vi "Sort channels.vi"(10 "Sort":T1[](array[typedef]), 11 "module datasets in":T2[](array[typedef])) -> (2 "Sort Out":T1[](array[typedef]), 3 "module datasets out":T2[](array[typedef]))   [LabVIEW 2015, in "GraphViz Mapping Visualizer.lvlib"]
doc: "Sorts all modules array by specified sort array. If sort array is smaller than module array, it will be padded with the first sort option in array."
uses:
  GraphViz Mapping Visualizer.lvlib
  <vilib>/NI/Tag Bus Module Framework/channel/TBM channel.lvclass
  <vilib>/NI/DCAF/Tag Editor Core/Configuration Editor/Classes/Engine Mappings/module information.ctl
  <vilib>/NI/DCAF/Tag Editor Core/Configuration Editor/Classes/Engine Mappings/Engine Mappings.lvclass
  Sort Options.ctl
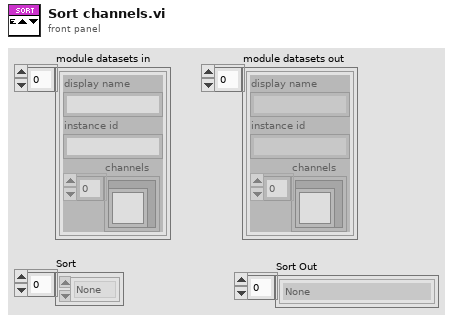
[diagram p1: front panel]
types:
  T1 = typedef "GraphViz Mapping Visualizer.lvlib/Sort Options.ctl" = enum16{"None", "All Ascending", "All Descending", "Channel Type Ascending", "Channel Type Descending"}
  T2 = typedef "PL Framework Configuration Tool.lvlib/Engine Mappings.lvclass/module information.ctl" = cluster{"display name":string, "instance id":string, "channels":refnum<class "TBM channel.lvclass">[]}
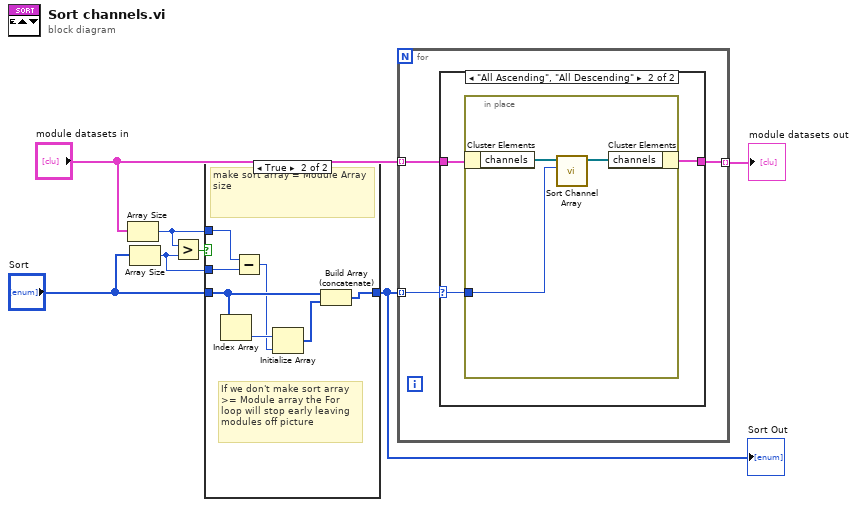
[diagram p0: block diagram]
diagram:
  n1 = Array Size(array="module datasets in") -> (size(s)=w2:i32)
  n2 = Array Size(array="Sort") -> (size(s)=w1:i32)
  n3 = Greater?(x=w2, y=w1) -> (0:w5:bool)
  n4 = case shown="True" w5 {
    tunnel: "Sort" -> [w8 w14]
    tunnel: [w8 w15] -> w3
    tunnel: w2 -> [_ w10]
    tunnel: w1 -> [_ w11]
    frame False {
    }
    frame True {
      # "If we don't make sort array\n>= Module array the For\nloop will stop early leaving\nmodules off picture"
      # "make sort array = Module Array size"
      n5 = Index Array(array=w14) -> (element=w13:T1)  [unwired: 1 in]
      n6 = Subtract(x=w10, y=w11) -> (x-y=w9:i32)
      n7 = Initialize Array(w13, w9) -> (w12:T1[])
      n8 = Build Array (concatenate)(w14, w12) -> (w15:T1[])
    }
  }
  "Sort Out" <- w3
  n9 = for {
    tunnel: w3 -> [w16] mode=indexing
    tunnel: [w18] -> w7 mode=indexing
    tunnel: "module datasets in" -> [w17] mode=indexing
    n10 = case shown="\"All Ascending\", \"All Descending\"" w16 {
      selector: w16 -> [_ w21]
      tunnel: w17 -> [w19 w22]
      tunnel: [w19 w20] -> w18
      frame "None", Default {
      }
      frame "All Ascending", "All Descending" {
        n11 = in-place {
          in-place-border: w21 -> [w24]
          n12 = in-place-cluster #1(w22) -> ("channels"=w25:refnum<class "TBM channel.lvclass">[])
          n13 = call "Sort Channel Array.vi"("Sort"=w24, "channels"=w25) -> ("Array"=w23:refnum<class "TBM channel.lvclass">[])  [unwired: 9 in]
          n14 = in-place-cluster #1("channels"=w23) -> (w20:T2)
        }
      }
    }
  }
  "module datasets out" <- w7
